vi "Read DAQ.vi"(8 "error in (no error)":errorcluster, 10 "Acq and Logging Props":T1, 11 "DAQmx Task Name":refnum<k21>) -> (0 "error out":errorcluster, 1 "Waveform Data":waveform(dbl)[](array[waveform]), 3 "Acq and Logging Props dup":T1)   [LabVIEW 2013]
doc: "Reads waveform data from the DAQmx device."
uses:
  <vilib>/DAQmx/read.llb/DAQmx Read (Analog 1D Wfm NChan NSamp).vi
  Globals - Monitoring Variables.vi
  <vilib>/DAQmx/miscellaneous.llb/DAQmx Fill In Error Info.vi
  <resource>/objmgr/daqmx.rc
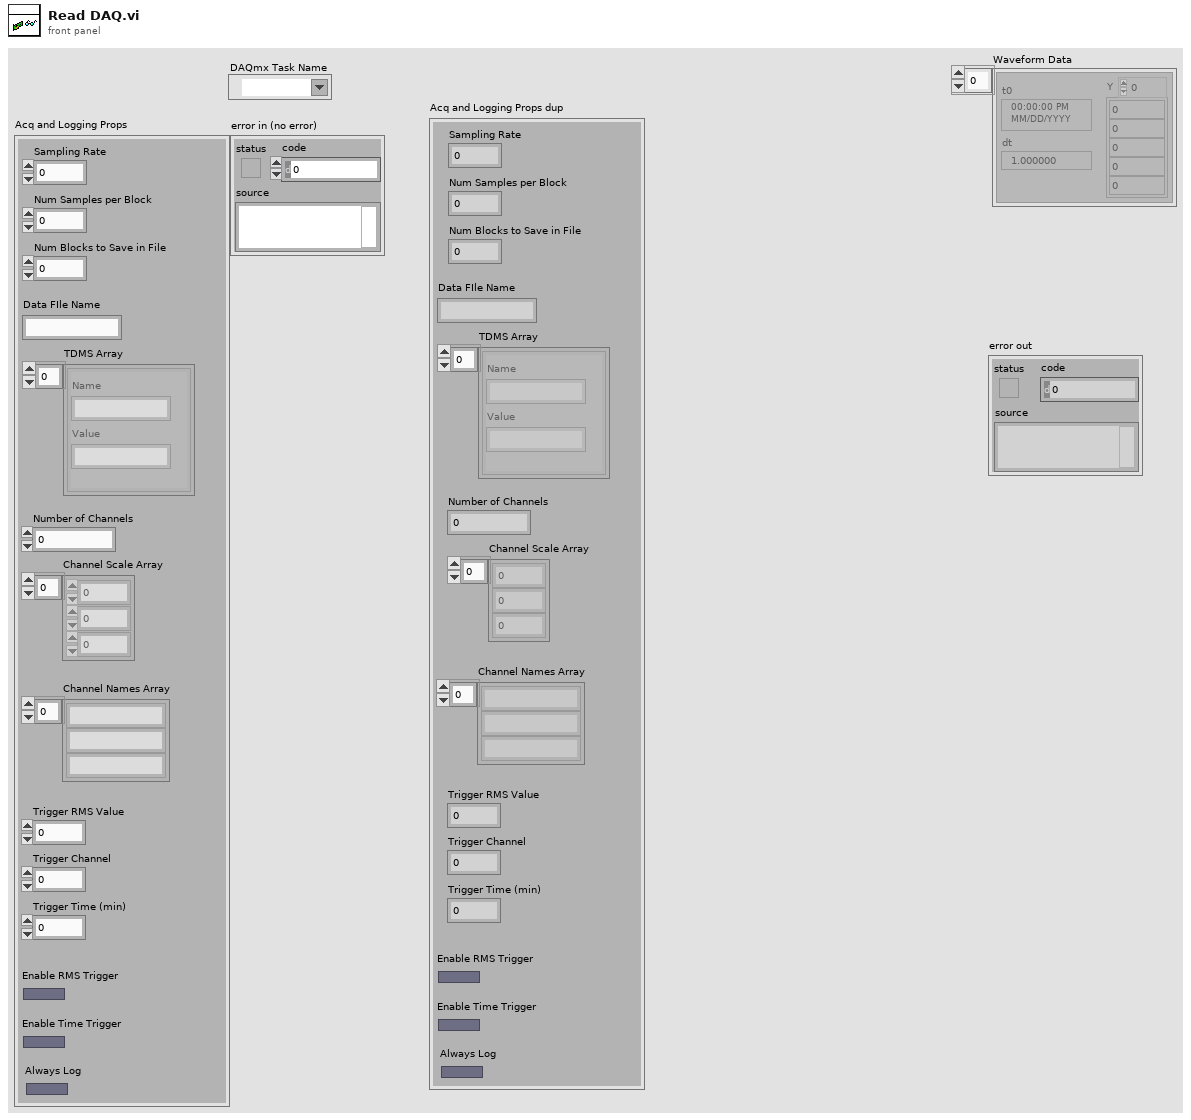
[diagram p1: front panel]
types:
  T1 = cluster{"Sampling Rate":dbl, "Num Samples per Block":i32, "Num Blocks to Save in File":i32, "Data FIle Name":string, "TDMS Array":cluster{"Name":string, "Value":string}[], "Number of Channels":i32, "Channel Scale Array":dbl[], "Channel Names Array":string[], "Trigger RMS Value":dbl, "Trigger Channel":i32, "Trigger Time (min)":i32, "Enable RMS Trigger":bool, "Enable Time Trigger":bool, "Always Log":bool}
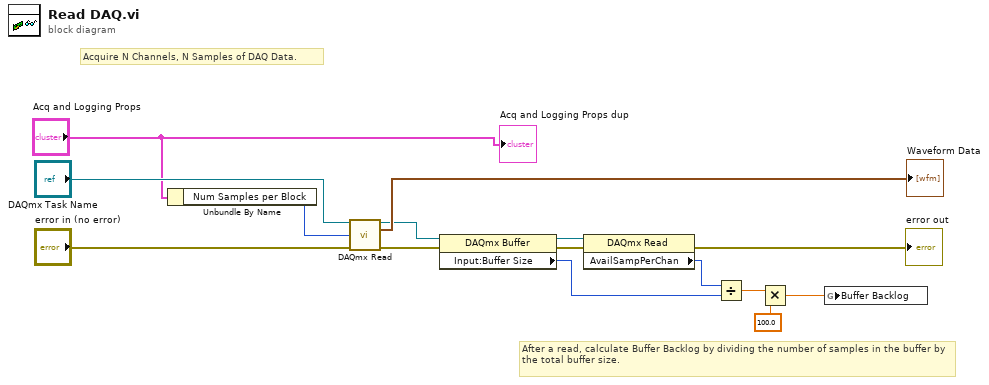
[diagram p0: block diagram]
diagram:
  # "After a read, calculate Buffer Backlog by dividing the number of samples in the buffer by the total buffer size."
  # "Acquire N Channels, N Samples of DAQ Data."
  n1 = Unbundle By Name("Acq and Logging Props") -> ("Num Samples per Block"=w14:i32)
  n2 = call-poly <vilib>:"DAQmx Read.vi"("task/channels in"="DAQmx Task Name", "number of samples per channel"=w14, "error in"="error in (no error)") -> ("task out"=w10:refnum<k21>, "data"=→"Waveform Data":waveform(dbl)[], "error out"=w11:errorcluster)  [unwired: 10 in]
  n3 = property class="DAQmx Buffer"(reference=w10, error in=w11) -> (reference out=w8:refnum<k21>, error out=w9:errorcluster, "Input:Buffer Size"=w7:u32)
  n4 = property class="DAQmx Read"(reference=w8, error in=w9) -> (error out=→"error out":errorcluster, "AvailSampPerChan"=w3:u32)  [unwired: 1 out]
  n5 = Divide(x=w3, y=w7) -> (x/y=w5:dbl)
  n6 = Multiply(x=w5, y=100.0) -> (x*y=w2:dbl)
  n7 = global write "Globals - Monitoring Variables.vi" "Buffer Backlog"(w2) -> ()
  "Acq and Logging Props dup" <- "Acq and Logging Props"
